vi "Fifo-Wait4Flag.vi"(8 "Raise Flag ?":bool, 11 "Ctl Refnum IN":refnum<vi>) -> (0 "Flag Value":bool, 3 "Ctl Refnum OUT":refnum<vi>)   [LabVIEW 2019]
panel:
  out "error out":errorcluster
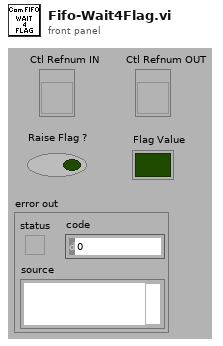
[diagram p1: front panel]
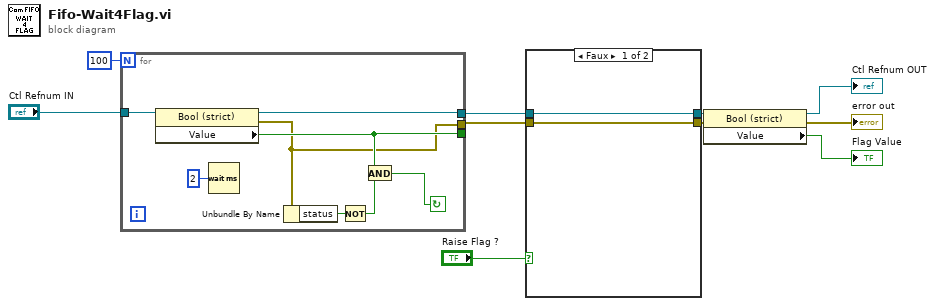
[diagram p0: block diagram]
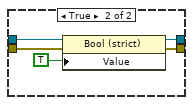
[diagram p2: hidden frame]
diagram:
  n1 = for {
    N: 100 -> [_]
    tunnel: "Ctl Refnum IN" -> [w18]
    tunnel: [w13] -> _
    tunnel: [w15] -> w9
    tunnel: [w12] -> w8
    stop <- w11 continue-if-true
    n2 = property on="Property Node" class="Bool (strict)"(reference=w18) -> (reference out=w15:refnum<vi>, error out=w12:errorcluster, "Value"=w13:bool)  [unwired: 1 in]
    n3 = Wait (ms)(milliseconds to wait=u32 2) -> ()  [unwired: 1 out]
    n4 = Unbundle By Name(w12) -> ("status"=w17:bool)
    n5 = Not(x=w17) -> (.not. x?=w16:bool)
    n6 = And(x=w13, y=w16) -> (x .and. y?=w11:bool)
  }
  n7 = case shown="Faux" "Raise Flag ?" {
    tunnel: w9 -> [w20 w25]
    tunnel: w8 -> [w19 w24]
    tunnel: [w20 w23] -> w6
    tunnel: [w19 w22] -> w5
    frame False {
    }
    frame True {
      n8 = property on="Property Node" class="Bool (strict)"(reference=w25, error in=w24, "Value"=TRUE) -> (reference out=w23:refnum<vi>, error out=w22:errorcluster)
    }
  }
  n9 = property on="Property Node" class="Bool (strict)"(reference=w6, error in=w5) -> (reference out=→"Ctl Refnum OUT":refnum<vi>, error out=→"error out":errorcluster, "Value"=→"Flag Value":bool)
